vi "TDMS Logger.vi"(6 "Duration(sec)":u16=1000, 8 "error in":errorcluster, 9 "Logging path":path, 10 "Socket":string, 11 "SequenceContext":refnum<k7>) -> (0 "Error Out":errorcluster, 3 "Change Fname?":bool)   [LabVIEW 2021]
doc: "This VI loops until either the Stop button is pressed or the calling TestStand sequence is terminated. The Termination Monitor VI allows this VI to query the TestStand execution for its current status."
uses:
  TDMS AE Control.ctl
  DataSet.ctl
panel:
  out "Logging?":bool
  out "Time":string="0  00:01:15"
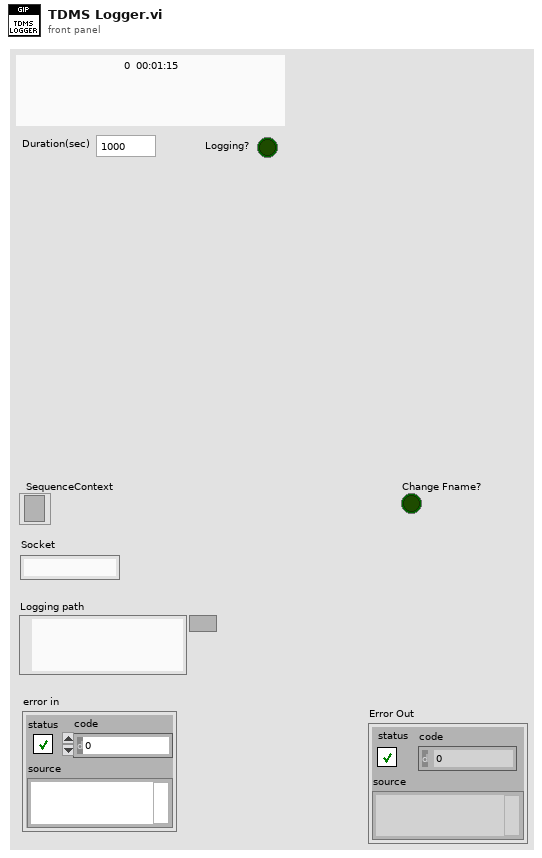
[diagram p1: front panel]
types:
  T1 = typedef "TDMS AE Control.ctl" = enum16{"Open", "Write", "Check Name", "Stop"}
  T2 = typedef "DataSet.ctl" = cluster{"Channel":string, "Data":dbl}
  T3 = typedef "TestStand - Status Monitor.ctl" = cluster{"Sequence Context":refnum<k7>, "Execution":refnum<k7>, "Termination Monitor":refnum<k7>}
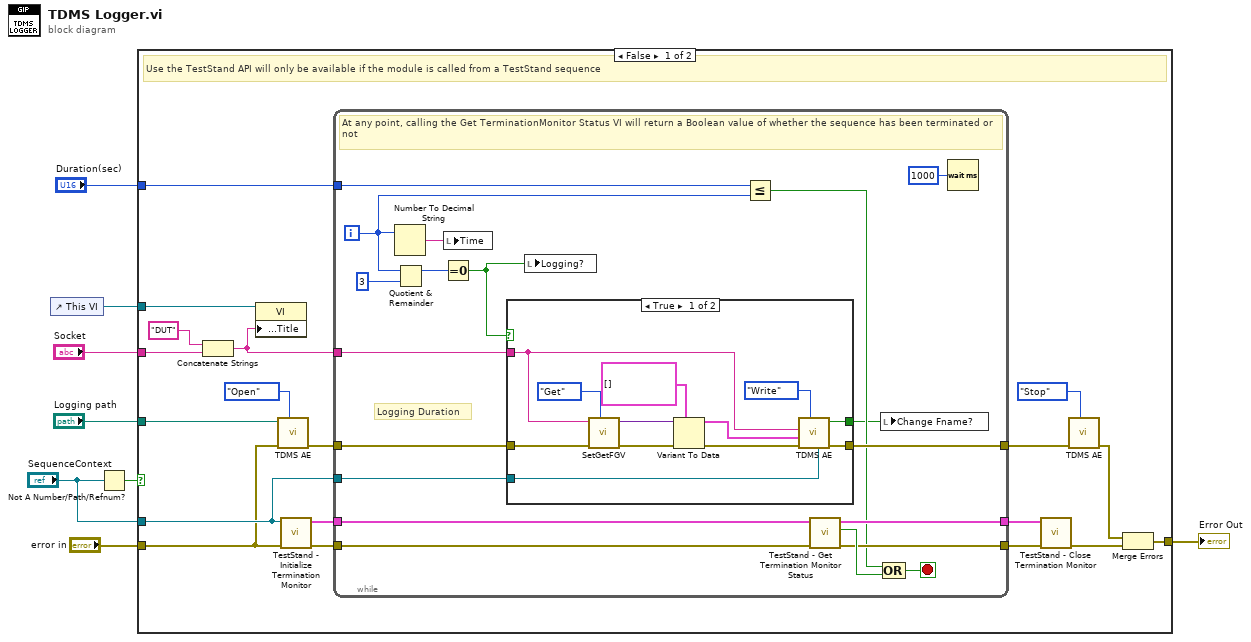
[diagram p0: block diagram]
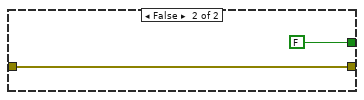
[diagram p2: hidden frame]
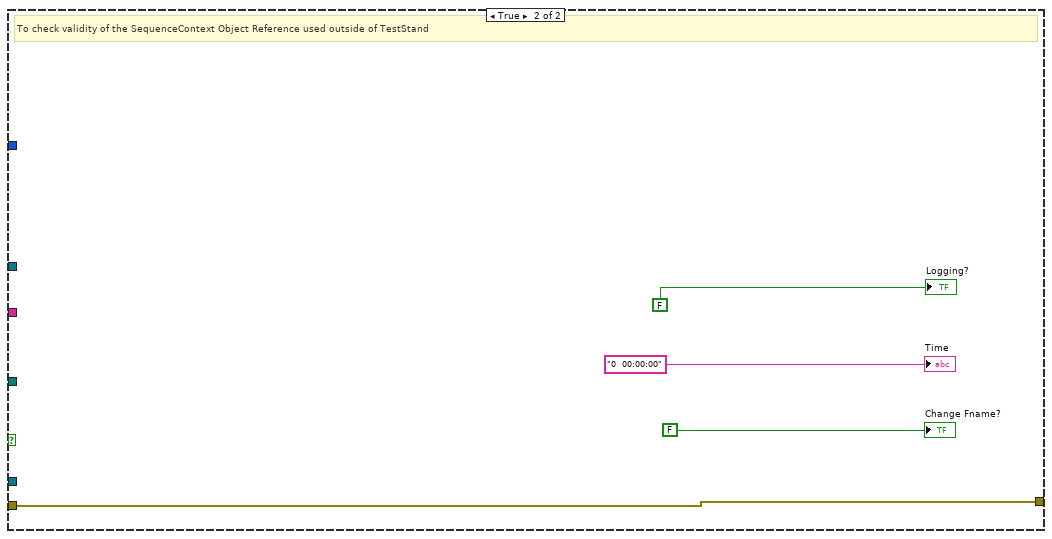
[diagram p3: hidden frame]
diagram:
  n1 = control-ref of="This VI"() -> (w1:refnum<vi>)
  n2 = Not A Number/Path/Refnum?(number/path/refnum="SequenceContext") -> (NaN/Path/Refnum?=w6:bool)
  n3 = case shown="False" w6 {
    tunnel: [w24 w64] -> w8
    tunnel: "error in" -> [w12 w64]
    tunnel: "SequenceContext" -> [w13 _]
    tunnel: "Logging path" -> [w16 _]
    tunnel: "Socket" -> [w11 _]
    tunnel: "Duration(sec)" -> [w15 _]
    tunnel: w1 -> [w14 _]
    frame False {
      # "Use the TestStand API will only be available if the module is called from a TestStand sequence"
      n4 = Concatenate Strings("DUT" ("string"), w11) -> (w10:string)
      n5 = property class="VI"(reference=w14, "Front Panel.Title"=w10) -> ()  [unwired: 1 in, 2 out]
      n6 = call "TDMS AE.vi"("Control"=TDMS_AE_Control."Open", "Error in"=w12, "Logging path"=w16) -> ("error out"=w19:errorcluster)  [unwired: 7 in, 1 out]
      n7 = call <vilib>:"TestStand - Initialize Termination Monitor.vi"("error in (no error)"=w12, "Sequence Context In"=w13) -> ("error out"=w27:errorcluster, "Status Monitor Out"=w26:T3)  [unwired: 8 in]
      n8 = while {
        tunnel: w26 -> [w46]
        tunnel: [w45] -> w22
        tunnel: w27 -> [w43]
        tunnel: [w41] -> w23
        tunnel: w19 -> [w38]
        tunnel: w10 -> [w33]
        tunnel: w15 -> [w36]
        tunnel: [w37] -> w17
        tunnel: w13 -> [w31]
        i -> [w35]
        stop <- w44 stop-if-true
        # "Logging Duration"
        # "At any point, calling the Get TerminationMonitor Status VI will return a Boolean value of whether the sequence has been terminated or not"
        n9 = Number To Decimal String(number=w35) -> (decimal integer string=w30:string)  [unwired: 1 in]
        n10 = Quotient & Remainder(x=w35, y=3) -> (x-y*floor(x/y)=w32:i32)  [unwired: 1 out]
        n11 = Equal To 0?(x=w32) -> (x = 0?=w29:bool)
        n12 = local write "Time"(w30) -> ()
        n13 = case shown="True" w29 {
          tunnel: [w57 FALSE ("Is Fname changed?")] -> w28
          tunnel: w38 -> [w54 w60]
          tunnel: [w56 w60] -> w37
          tunnel: w33 -> [w47 _]
          tunnel: w31 -> [w55 _]
          frame True {
            n14 = call "SetGetFGV.vi"("Method (Get)"=enum16{"Get", "Set"}."Get", "error in"=w54, "FGVname"=w47) -> ("error out"=w53:errorcluster, "Data out"=w50:variant)  [unwired: 7 in]
            n15 = Variant To Data(error in=w53, type=T2[] [] ("Channels"), Variant=w50) -> (data=w48:T2[], error out=w51:errorcluster)
            n16 = call "TDMS AE.vi"("Context"=w55, "Control"=TDMS_AE_Control."Write", "Error in"=w51, "Channels"=w48, "Group Name"=w47) -> ("error out"=w56:errorcluster, "Is Fname changed?"=w57:bool)  [unwired: 5 in]
          }
          frame False {
          }
        }
        n17 = local write "Logging?"(w29) -> ()
        n18 = Less Or Equal?(x=w36, y=w35) -> (x <= y?=w34:bool)
        n19 = call <vilib>:"TestStand - Get Termination Monitor Status.vi"("error in (no error)"=w43, "Status Monitor In"=w46) -> ("error out"=w41:errorcluster, "Terminating or Aborting"=w42:bool, "Status Monitor Out"=w45:T3)  [unwired: 7 in]
        n20 = local write "Change Fname?"(w28) -> ()
        n21 = Compound Arithmetic op=OR(w34, w42) -> (w44:bool)
        n22 = Wait (ms)(milliseconds to wait=u32 1000) -> ()  [unwired: 1 out]
      }
      n23 = call <vilib>:"TestStand - Close Termination Monitor.vi"("error in (no error)"=w23, "Status Monitor In"=w22) -> ("error out"=w25:errorcluster)  [unwired: 9 in]
      n24 = call "TDMS AE.vi"("Control"=TDMS_AE_Control."Stop", "Error in"=w17) -> ("error out"=w21:errorcluster)  [unwired: 8 in, 1 out]
      n25 = Merge Errors(w21, w25) -> (w24:errorcluster)
    }
    frame True {
      # "To check validity of the SequenceContext Object Reference used outside of TestStand"
      "Time" <- "0  00:00:00" ("Time")
      "Logging?" <- FALSE ("Logging?")
      "Change Fname?" <- FALSE ("Change Fname?")
    }
  }
  "Error Out" <- w8
